vi "contFFLoop.vi"(7 "error in (no error)":errorcluster, 9 "activate":u8) -> (0 "error out":errorcluster)   [LabVIEW 2015, in "ESLSCDLL.lvlib"]
uses:
  ESLSCDLL.lvlib
  Globals.vi
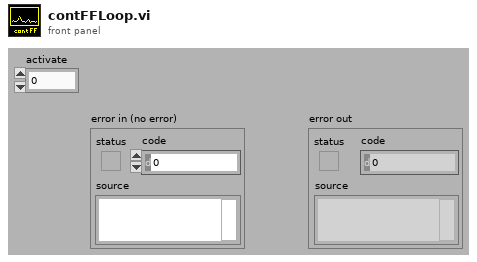
[diagram p1: front panel]
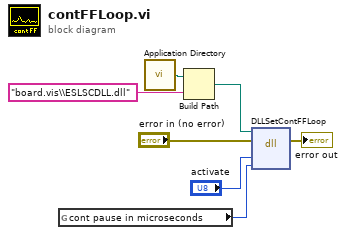
[diagram p0: block diagram]
diagram:
  n1 = global read "Globals.vi" "cont pause in microseconds"() -> (w4:u32)
  n2 = call <vilib>:"Application Directory.vi"() -> ("Application Directory"=w3:path)
  n3 = Build Path(base path=w3, name or relative path="board.vis\\ESLSCDLL.dll") -> (appended path=w1:path)
  n4 = dll-call lib="C:/ENTW/PCIE/LV64/board.vis/ESLSCDLL.dll" fn="DLLSetContFFLoop"(path in=w1, error in="error in (no error)", "activate"="activate", "pause"=w4) -> (error out=→"error out":errorcluster)  [unwired: 4 in, 1 out]
